vi "Search Sysdef for Targets.vi"(8 "error in (no error)":errorcluster, 11 "NIVS.System Definition Root":refnum<k24>) -> (0 "error out":errorcluster, 1 "Target Names":string[](array[string]), 3 "NIVS.System Defintion Root Out":refnum<k24>, 7 "Target Nodes":refnum<k24>[](array[refnum]))   [LabVIEW 2020, in "Instrument Workspace Shared.lvlib"]
uses:
  Instrument Workspace Shared.lvlib
  NationalInstruments.VeriStand.SystemStorage
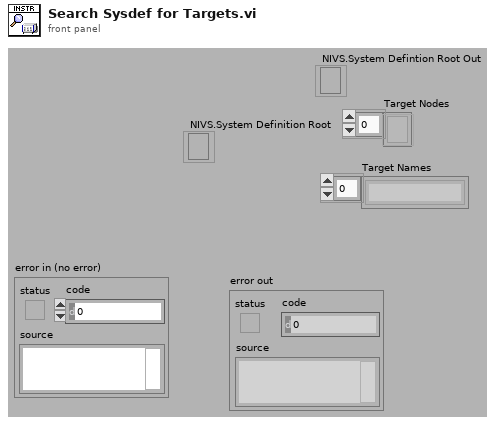
[diagram p1: front panel]
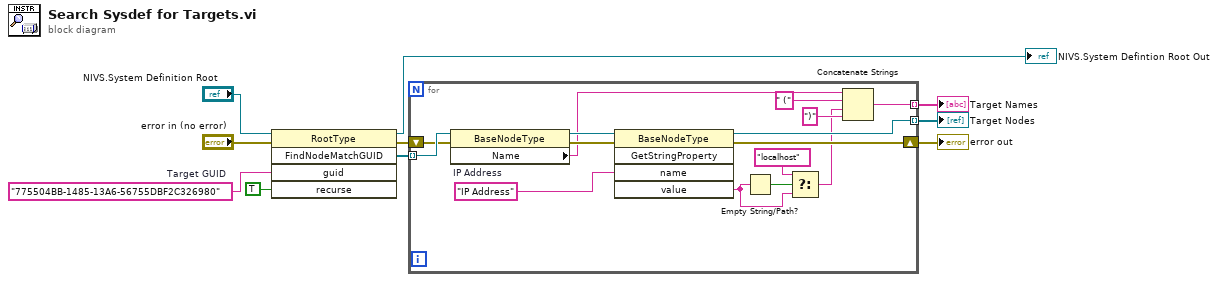
[diagram p0: block diagram]
diagram:
  w4 = "775504BB-1485-13A6-56755DBF2C326980"  # Target GUID
  n1 = invoke class="RootType" method="FindNodeMatchGUID"(reference="NIVS.System Definition Root", error in="error in (no error)", "guid"=w4, "recurse"=TRUE) -> (reference out=→"NIVS.System Defintion Root Out":refnum<k24>, error out=w2:errorcluster, "FindNodeMatchGUID"=w3:refnum<k24>[])  [unwired: 1 in, 2 out]
  n2 = for {
    tunnel: w3 -> [w25] mode=indexing
    shift-right: [w21] -> w5
    shift-left: w2 -> [w24]
    tunnel: [w20] -> w7 mode=indexing
    tunnel: [w15] -> w6 mode=indexing
    w19 = "IP Address"  # IP Address
    n3 = property class="BaseNodeType"(reference=w25, error in=w24) -> (reference out=w23:refnum<k24>, error out=w22:errorcluster, "Name"=w16:string)
    n4 = invoke class="BaseNodeType" method="GetStringProperty"(reference=w23, error in=w22, "name"=w19) -> (reference out=w20:refnum<k24>, error out=w21:errorcluster, "value"=w12:string)  [unwired: 2 in, 2 out]
    n5 = Empty String/Path?(string/path=w12) -> (empty?=w14:bool)
    n6 = Select(t="localhost", s=w14, f=w12) -> (s? t:f=w11:string)
    n7 = Concatenate Strings(w16, " (" ("string"), w11, ")" ("string")) -> (w15:string)
  }
  "error out" <- w5
  "Target Nodes" <- w7
  "Target Names" <- w6
